vi "Data File Processing UI Message Queue.vi"(0 "msg type":T2, 7 "msg data":variant, 11 "error in":errorcluster) -> (4 "queue out":refnum<queue>, 15 "error out":errorcluster)   [LabVIEW 2012]
uses:
  Data File Processing UI Message Define.ctl
  Data File Processing UI Message Type Define.ctl
panel:
  in  "msg def":T1
  # "Input Data"
  # "Local Data"
  # "Output Data"
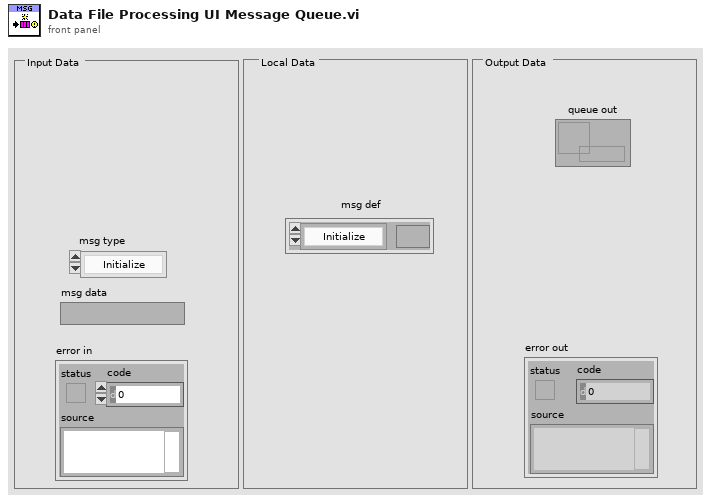
[diagram p1: front panel]
types:
  T1 = typedef "Data File Processing UI Message Define.ctl" = cluster{"data":variant, "type":T2}
  T2 = typedef "Data File Processing UI Message Type Define.ctl" = enum32{"Initialize", "SleepThread", "ErrorHandler", "NoEvent", "PreExit", "Exit", "----Action----", "OpenFile", "ReadAllCompute", "SaveFile", "RedrawGraph", "SelectChannel"}
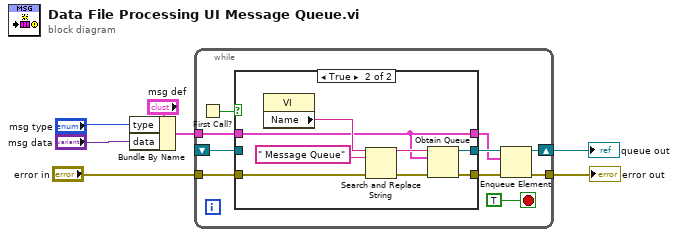
[diagram p0: block diagram]
diagram:
  n1 = Bundle By Name(cluster="msg def", "type"="msg type", "data"="msg data") -> (w1:T1)
  n2 = while {
    tunnel: "error in" -> [w17]
    tunnel: [w14] -> w6
    tunnel: w1 -> [w12]
    shift-right: [w15] -> w7
    shift-left: _ -> [w11]
    stop <- TRUE stop-if-true
    n3 = First Call?() -> (First Call?: T/F=w10:bool)
    n4 = case shown="True" w10 {
      tunnel: w17 -> [w19 w27]
      tunnel: [w19 w26] -> w16
      tunnel: [w20 w25] -> w13
      tunnel: w12 -> [w18 w21]
      tunnel: w11 -> [w20 _]
      tunnel: [w18 w21] -> w9
      frame False {
      }
      frame True {
        n5 = property class="VI"() -> ("Name"=w24:string)  [unwired: 2 in, 2 out]
        n6 = Search and Replace String(input string=w24, search string=" Message Queue") -> (result string=w23:string)  [unwired: 6 in, 3 out]
        n7 = Obtain Queue(name (unnamed)=w23, element data type=w21, error in (no error)=w27) -> (queue out=w25:refnum<queue>, error out=w26:errorcluster)  [unwired: 2 in, 1 out]
      }
    }
    n8 = Enqueue Element(queue=w13, element=w9, error in (no error)=w16) -> (queue out=w15:refnum<queue>, error out=w14:errorcluster)  [unwired: 2 out]
  }
  "error out" <- w6
  "queue out" <- w7
